vi "Server Panel.vi"(8 "error in":errorcluster, 11 "server session ref":variant) -> (0 "error out":errorcluster, 3 "server session ref out":variant)   [LabVIEW 2018]
doc: "This is panel of TWM server. When the server is running, a client can connect to the created named pipe and control some of the TWM function via the pipe. This panel must be opened to keep the server alive!"
uses:
  Server Session Reference.ctl
  Server Session.ctl
  varilib/SGUI Assign References Mode.ctl
  Server Event.ctl
  Server Client Request.ctl
  Server Event Command.ctl
  varilib/SGUI Assign Multiple Strings With Tags By Label.vi
  varilib/varilib.lvlib
panel:
  out "srv session":T1
  out "server":i32
  in  "btn srv exit":bool
  out "str last data":string caption="Last command data"
  out "str last cmd":string caption="Last command header"
  out "led run":bool caption="Running"
  in  "btn srv stop":bool
  in  "btn srv start":bool
  in  "pipe name":string="\\\\.\\pipe\\TWM:server" caption="Named Pipe Identifier"
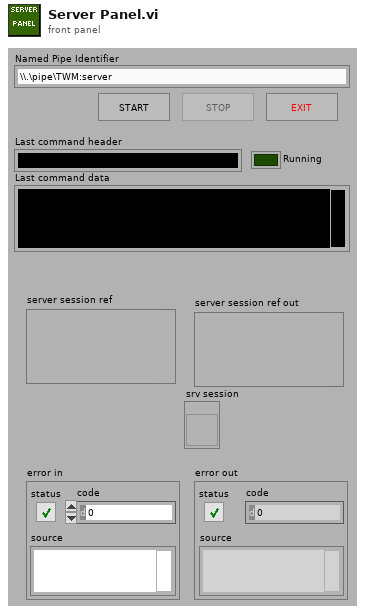
[diagram p1: front panel]
types:
  T1 = typedef "Server Session Reference.ctl" = refnum<vi>
  T2 = typedef "varilib.lvlib/SGUI Assign References Mode.ctl" = enum16{"Add to stack", "Overwrite", "Release last", "Release ID"}
  T3 = typedef "Server Session.ctl" = cluster{"cmd event":variant, "answer event":variant}
  T4 = typedef "Server Event.ctl" = cluster{"client request":T5, "command":T6}
  T5 = typedef "Server Client Request.ctl" = cluster{"info data":string, "answer handle":i32}
  T6 = typedef "Server Event Command.ctl" = enum16{"None", "Restart", "Identify", "Set measurement", "Start", "Get status", "Get result", "Stop", "Set corrections", "Get algorithm info"}
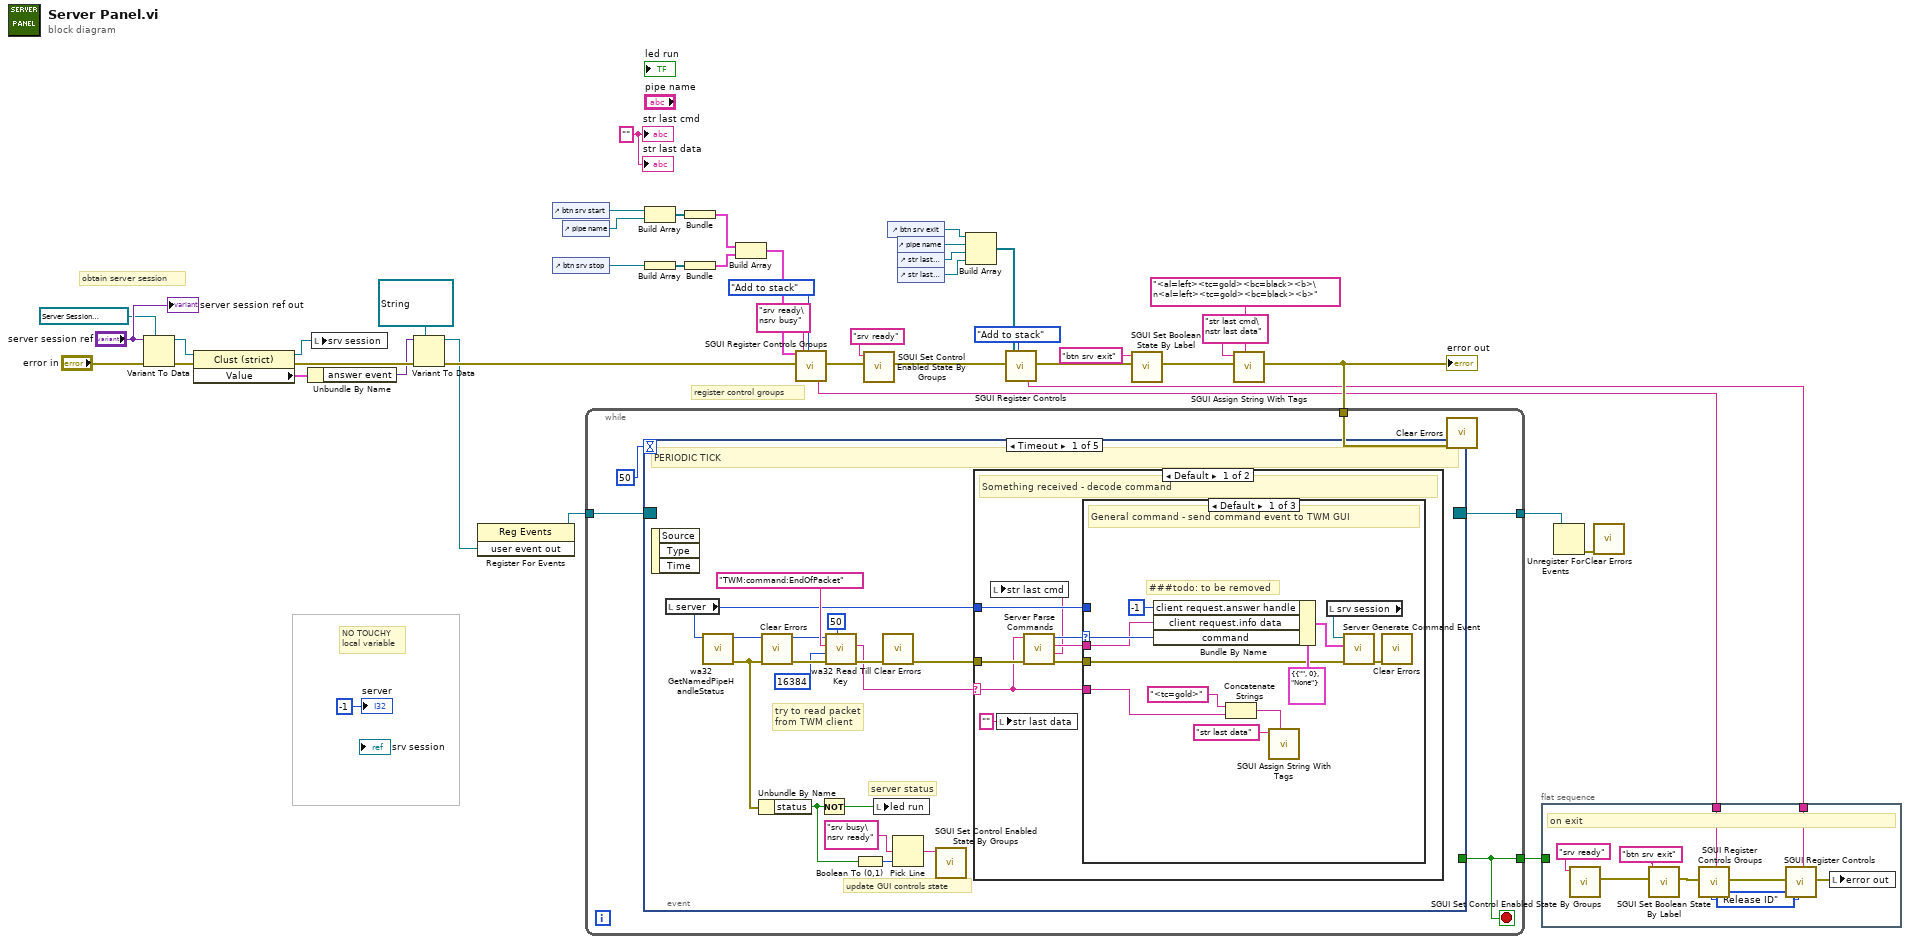
[diagram p0: block diagram]
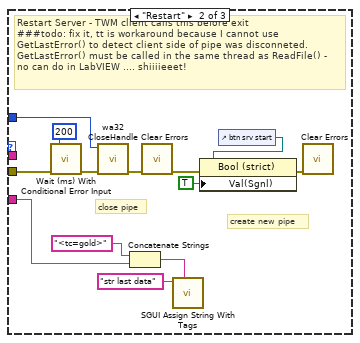
[diagram p2: hidden frame]
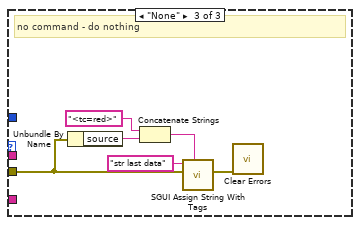
[diagram p3: hidden frame]
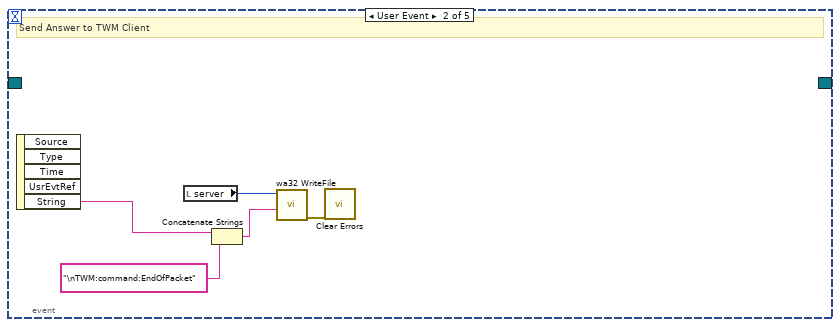
[diagram p5: hidden frame]
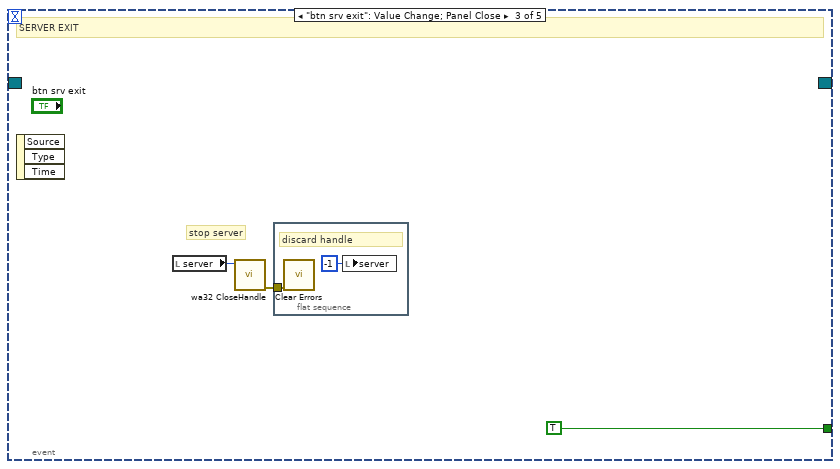
[diagram p6: hidden frame]
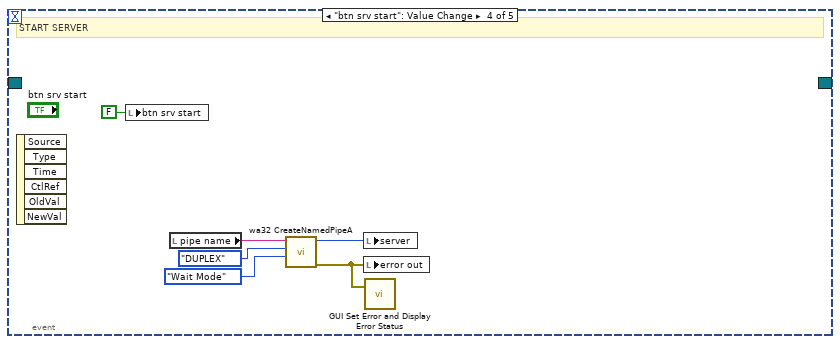
[diagram p7: hidden frame]
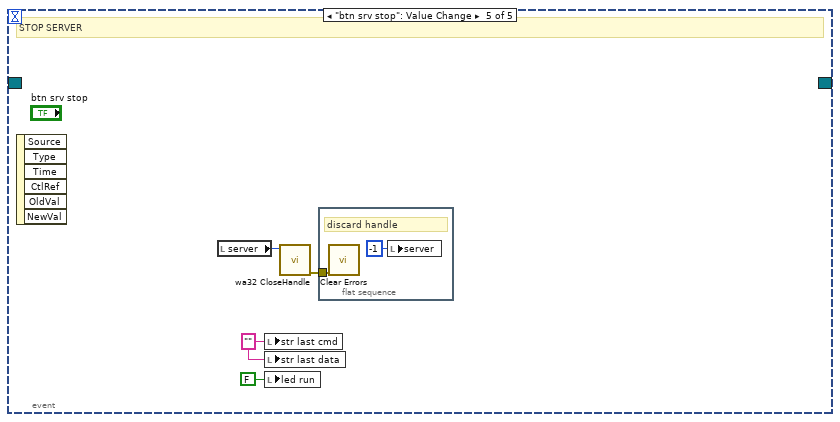
[diagram p8: hidden frame]
diagram:
  w23 = "" ("str last cmd")
  # "obtain server session"
  # "NO TOUCHY\nlocal variable"
  # "register control groups"
  n1 = Variant To Data(error in="error in", type=T1 refnum ("server ref"), Variant="server session ref") -> (data=w14:T1, error out=w15:errorcluster)
  n2 = property class="Clust (strict)"(reference=w14, error in=w15) -> (reference out=w13:T1, error out=w11:errorcluster, "Value"=w12:T3)
  n3 = Unbundle By Name(w12) -> ("answer event"=w9:variant)
  n4 = local write "srv session"(w13) -> ()
  n5 = Variant To Data(error in=w11, type=refnum<user-event> refnum ("user event out"), Variant=w9) -> (data=w7:refnum<user-event>, error out=w10:errorcluster)
  n6 = register-events(w7) -> (reference out=w16:refnum<event-registration>)  [unwired: 2 in, 1 out]
  n7 = control-ref of="btn srv start"() -> (w40:refnum<vi>)
  n8 = control-ref of="btn srv stop"() -> (w41:refnum<vi>)
  n9 = control-ref of="pipe name"() -> (w39:refnum<vi>)
  n10 = Build Array(w40, w39) -> (w44:refnum<vi>[])
  n11 = Build Array(w41) -> (w42:refnum<vi>[])
  n12 = Bundle(w44) -> (w45:cluster{refnum<vi>[]})  [unwired: 1 in]
  n13 = Bundle(w42) -> (w43:cluster{refnum<vi>[]})  [unwired: 1 in]
  n14 = Build Array(w45, w43) -> (w38:cluster{refnum<vi>[]}[])
  n15 = call "SGUI Register Controls Groups.vi"("control groups"=w38, "error in"=w10, "groups names"="srv ready\nsrv busy", "register mode (overwrite)"=SGUI_Assign_References_Mode."Add to stack") -> ("assigned ID"=w19:string, "error out"=w35:errorcluster)  [unwired: 14 in]
  n16 = call "SGUI Set Control Enabled State By Groups.vi"("error in"=w35, "group name to enable (none)"="srv ready") -> ("error out"=w32:errorcluster)  [unwired: 8 in, 1 out]
  n17 = control-ref of="btn srv exit"() -> (w1:refnum<vi>)
  n18 = control-ref of="pipe name"() -> (w31:refnum<vi>)
  n19 = control-ref of="str last cmd"() -> (w30:refnum<vi>)
  n20 = control-ref of="str last data"() -> (w29:refnum<vi>)
  n21 = Build Array(w1, w31, w30, w29) -> (w28:refnum<vi>[])
  n22 = call "SGUI Register Controls.vi"("error in"=w32, "control references (empty)"=w28, "register mode (overwrite)"=SGUI_Assign_References_Mode."Add to stack") -> ("assigned ID"=w18:string, "error out"=w4:errorcluster)  [unwired: 14 in, 1 out]
  n23 = call "SGUI Set Boolean State By Label.vi"("error in"=w4, "control label(s) ('btn stop')"="btn srv exit" ("labels (empty)")) -> ("error out"=w3:errorcluster)  [unwired: 8 in, 1 out]
  n24 = call-poly "SGUI Assign String With Tags.vi"("error in"=w3, "label(s) (empty)"="str last cmd\nstr last data", "string (empty)"="<al=left><tc=gold><bc=black><b>\n<al=left><tc=gold><bc=black><b>") -> ("error out"=w24:errorcluster)  [unwired: 7 in, 1 out]
  "error out" <- w24
  n25 = while {
    tunnel: w24 -> [w49]
    tunnel: [w48] -> w33
    tunnel: w16 -> [w47]
    tunnel: [w46] -> w6
    stop <- w48 stop-if-true
    n26 = event shown="[0] Timeout" {
      selector: w47 -> [_ _ _ _ _]
      dyn-events: [_ _ _ _ _] -> w46
      timeout: 50 -> [_ _ _ _ _]
      tunnel: [_ _ TRUE _ _] -> w48
      event Timeout {
        # "try to read packet\nfrom TWM client"
        # "server status"
        # "update GUI controls state"
        # "PERIODIC TICK"
        n27 = event-data() -> ()  [unwired: 1 in, 3 out]
        n28 = local read "server"() -> (w52:i32)
        n29 = call "wa32 GetNamedPipeHandleStatus.vi"("handle"=w52) -> ("error out"=w57:errorcluster, "handle out"=w53:i32)  [unwired: 7 in, 2 out]
        n30 = Unbundle By Name(w57) -> ("status"=w59:bool)
        n31 = call <vilib>:"Clear Errors.vi"("error in (no error)"=w57) -> ("error out"=w54:errorcluster)  [unwired: 5 in, 1 out]
        n32 = Not(x=w59) -> (.not. x?=w63:bool)
        n33 = call "wa32 Read Till Key.vi"("timeout [ms] (1000)"=50, "error in"=w54, "max message length (1024)"=16384, "key string"="TWM:command:EndOfPacket", "handle"=w53) -> ("error out"=w64:errorcluster, "read message"=w56:string)  [unwired: 4 in, 1 out]
        n34 = Boolean To (0,1)(Boolean=w59) -> (0, 1=w62:i16)
        n35 = local write "led run"(w63) -> ()
        n36 = call <vilib>:"Clear Errors.vi"("error in (no error)"=w64) -> ("error out"=w55:errorcluster)  [unwired: 5 in, 1 out]
        n37 = Pick Line(multi-line string="srv busy\nsrv ready", line index=w62) -> (output string=w60:string)  [unwired: 1 in]
        n38 = call "SGUI Set Control Enabled State By Groups.vi"("group name to enable (none)"=w60) -> ()  [unwired: 9 in, 2 out]
        n39 = case shown="Default" w56 {
          selector: w56 -> [w67 _]
          tunnel: w55 -> [w73 _]
          tunnel: w52 -> [w70 _]
          frame Default {
            # "Something received - decode command"
            n40 = local write "str last data"("" ("str last data")) -> ()
            n41 = call "Server Parse Commands.vi"("error in"=w73, "string"=w67) -> ("error out"=w71:errorcluster, "command string"=w66:string, "command data"=w69:string, "command"=w72:T6)  [unwired: 6 in]
            n42 = local write "str last cmd"(w66) -> ()
            n43 = case shown="Default" w72 {
              selector: w72 -> [w80 _ _]
              tunnel: w71 -> [w81 w93 w102]
              tunnel: w70 -> [_ w98 _]
              tunnel: w69 -> [w74 _ _]
              tunnel: w67 -> [w75 w86 _]
              frame Default {
                # "###todo: to be removed"
                # "General command - send command event to TWM GUI"
                n44 = Bundle By Name(cluster=T4 {"client request"={"info data"="", "answer handle"=0}, "command"=enum."None"} ("event data"), "client request.answer handle"=-1, "client request.info data"=w74, "command"=w80) -> (w82:T4)
                n45 = Concatenate Strings("<tc=gold>" ("string"), w75) -> (w77:string)
                n46 = call-poly "SGUI Assign String With Tags.vi"("label(s) (empty)"="str last data", "string (empty)"=w77) -> ()  [unwired: 8 in, 2 out]
                n47 = local read "srv session"() -> (w84:T1)
                n48 = call "Server Generate Command Event.vi"("error in"=w81, "event data"=w82, "server event ref"=w84) -> ("error out"=w85:errorcluster)  [unwired: 8 in]
                n49 = call <vilib>:"Clear Errors.vi"("error in (no error)"=w85) -> ()  [unwired: 5 in, 2 out]
              }
              frame "Restart" {
                # "create new pipe"
                # "close pipe"
                # "Restart Server - TWM client calls this before exit\n###todo: fix it, tt is workaround because I cannot use\nGetLastError() to detect client side of pipe was disconneted.\nGetLastError() must be called in the same thread as ReadFile() - \nno can do in LabVIEW .... shiiiieeet!"
                n50 = call "Wait (ms) With Conditional Error Input.vi"("error in (no error)"=w93, "milliseconds to wait"=u32 200) -> ("error out"=w92:errorcluster)  [unwired: 8 in, 1 out]
                n51 = call "wa32 CloseHandle.vi"("error in"=w92, "handle"=w98) -> ("error out"=w97:errorcluster)  [unwired: 9 in]
                n52 = Concatenate Strings("<tc=gold>" ("string"), w86) -> (w88:string)
                n53 = call <vilib>:"Clear Errors.vi"("error in (no error)"=w97) -> ("error out"=w90:errorcluster)  [unwired: 5 in, 1 out]
                n54 = call-poly "SGUI Assign String With Tags.vi"("label(s) (empty)"="str last data", "string (empty)"=w88) -> ()  [unwired: 8 in, 2 out]
                n55 = control-ref of="btn srv start"() -> (w96:refnum<vi>)
                n56 = property class="Bool (strict)"(reference=w96, error in=w90, "Val(Sgnl)"=TRUE) -> (error out=w94:errorcluster)  [unwired: 1 out]
                n57 = call <vilib>:"Clear Errors.vi"("error in (no error)"=w94) -> ()  [unwired: 5 in, 2 out]
              }
              frame "None" {
                # "no command - do nothing"
                n58 = Unbundle By Name(w102) -> ("source"=w101:string)
                n59 = Concatenate Strings("<tc=red>" ("string"), w101) -> (w100:string)
                n60 = call-poly "SGUI Assign String With Tags.vi"("error in"=w102, "label(s) (empty)"="str last data", "string (empty)"=w100) -> ("error out"=w104:errorcluster)  [unwired: 7 in, 1 out]
                n61 = call <vilib>:"Clear Errors.vi"("error in (no error)"=w104) -> ()  [unwired: 5 in, 2 out]
              }
            }
          }
          frame "" {
          }
        }
      }
      event User Event {
        # "Send Answer to TWM Client"
        n62 = event-data() -> ("String"=w108:string)  [unwired: 1 in, 4 out]
        n63 = local read "server"() -> (w109:i32)
        n64 = Concatenate Strings(w108, "\nTWM:command:EndOfPacket" ("key string")) -> (w106:string)
        n65 = call "wa32 WriteFile.vi"("string data (empty)"=w106, "handle"=w109) -> ("error out"=w105:errorcluster)  [unwired: 7 in, 2 out]
        n66 = call <vilib>:"Clear Errors.vi"("error in (no error)"=w105) -> ()  [unwired: 5 in, 2 out]
      }
      event "btn srv exit": Value Change; Panel Close {
        # "stop server"
        # "SERVER EXIT"
        n67 = event-data() -> ()  [unwired: 1 in, 3 out]
        n68 = local read "server"() -> (w111:i32)
        n69 = call "wa32 CloseHandle.vi"("handle"=w111) -> ("error out"=w110:errorcluster)  [unwired: 10 in]
        n70 = flat-sequence {
          tunnel: w110 -> [w114]
          frame #0 {
            # "discard handle"
            n71 = call <vilib>:"Clear Errors.vi"("error in (no error)"=w114) -> ()  [unwired: 5 in, 2 out]
            n72 = local write "server"(-1 ("server")) -> ()
          }
        }
      }
      event "btn srv start": Value Change {
        # "START SERVER"
        n73 = event-data() -> ()  [unwired: 1 in, 6 out]
        n74 = local write "btn srv start"(FALSE ("btn srv start")) -> ()
        n75 = local read "pipe name"() -> (w120:string)
        n76 = call "wa32 CreateNamedPipeA.vi"("pipe mode"=enum16{"Wait Mode", "No Wait Mode"}."Wait Mode", "open mode"=enum16{"INBOUND", "OUTBOUND", "DUPLEX"}."DUPLEX", "file path"=w120) -> ("error out"=w116:errorcluster, "handle"=w117:i32)  [unwired: 7 in]
        n77 = local write "server"(w117) -> ()
        n78 = local write "error out"(w116) -> ()
        n79 = call "GUI Set Error and Display Error Status.vi"("error in"=w116) -> ()  [unwired: 4 in]
      }
      event "btn srv stop": Value Change {
        w122 = "" ("str last cmd")
        # "STOP SERVER"
        n80 = event-data() -> ()  [unwired: 1 in, 6 out]
        n81 = local read "server"() -> (w124:i32)
        n82 = local write "str last cmd"(w122) -> ()
        n83 = local write "str last data"(w122) -> ()
        n84 = local write "led run"(FALSE ("led run")) -> ()
        n85 = call "wa32 CloseHandle.vi"("handle"=w124) -> ("error out"=w123:errorcluster)  [unwired: 10 in]
        n86 = flat-sequence {
          tunnel: w123 -> [w126]
          frame #0 {
            # "discard handle"
            n87 = call <vilib>:"Clear Errors.vi"("error in (no error)"=w126) -> ()  [unwired: 5 in, 2 out]
            n88 = local write "server"(-1 ("server")) -> ()
          }
        }
      }
    }
    n89 = call <vilib>:"Clear Errors.vi"("error in (no error)"=w49) -> ()  [unwired: 5 in, 2 out]
  }
  n90 = flat-sequence {
    tunnel: w33 -> [_]
    tunnel: w19 -> [w131]
    tunnel: w18 -> [w130]
    frame #0 {
      w132 = SGUI_Assign_References_Mode."Release ID" ("register mode (overwrite)")
      # "on exit"
      n91 = call "SGUI Set Control Enabled State By Groups.vi"("group name to enable (none)"="srv ready") -> ("error out"=w128:errorcluster)  [unwired: 9 in, 1 out]
      n92 = call "SGUI Set Boolean State By Label.vi"("error in"=w128, "control label(s) ('btn stop')"="btn srv exit" ("labels (empty)")) -> ("error out"=w127:errorcluster)  [unwired: 8 in, 1 out]
      n93 = call "SGUI Register Controls Groups.vi"("error in"=w127, "register mode (overwrite)"=w132, "controls ID (empty)"=w131) -> ("error out"=w134:errorcluster)  [unwired: 15 in, 1 out]
      n94 = call "SGUI Register Controls.vi"("error in"=w134, "register mode (overwrite)"=w132, "controls ID (empty)"=w130) -> ("error out"=w133:errorcluster)  [unwired: 14 in, 2 out]
      n95 = local write "error out"(w133) -> ()
    }
  }
  n96 = Unregister For Events(event registration refnum=w6) -> (error out=w5:errorcluster)  [unwired: 1 in]
  n97 = call <vilib>:"Clear Errors.vi"("error in (no error)"=w5) -> ()  [unwired: 5 in, 2 out]
  "str last cmd" <- w23
  "str last data" <- w23
  "server" <- -1 ("server")
  "server session ref out" <- "server session ref"
